vi "MEASure_FETCh_READ.vi"(4 "Timeout (ms)":u32=1000, 5 "Sleep":bool, 6 "Digits":u8=5 min=1 max=5 step=1, 7 "Function":enum16{"MEASure", "READ", "FETCh"}(ring), 8 "Error in (no error)":errorcluster, 9 "Size":u16=1 min=1 max=4096 step=1, 10 "Select":T1={"X"=FALSE, "Y"=TRUE, "Z"=FALSE, "Temp"=FALSE, "Timstamp"=FALSE}, 11 "VISA resource":refnum<visa-resource-name>) -> (0 "Error out":errorcluster, 2 "Output":T2 {"Z" format="%.5f"; "Y" format="%.5f"; "X" format="%.5f"}, 3 "Dup VISA resource":refnum<visa-resource-name>)   [LabVIEW 2010]
doc: "Copyright (c) 2012 Metrolab Technology SA, Plan-les-Ouates, Geneva, Switzerland\nPerforms a measurement and parses the result."
panel:
  # "MEASure_FETCh_READ"
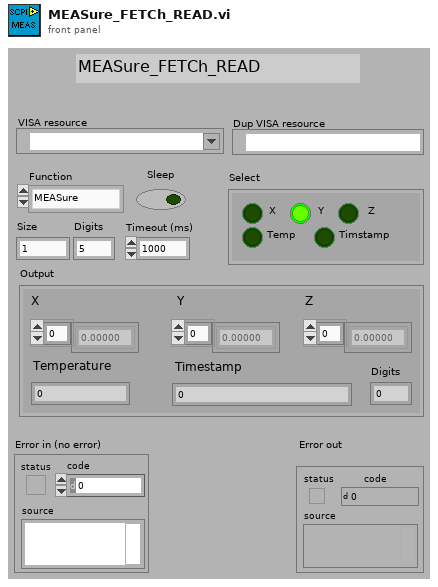
[diagram p1: front panel]
types:
  T1 = cluster{"X":bool, "Y":bool, "Z":bool, "Temp":bool, "Timstamp":bool}
  T2 = cluster{"X":dbl[], "Y":dbl[], "Z":dbl[], "Temperature":u16, "Timestamp":ext, "Digits":u8}
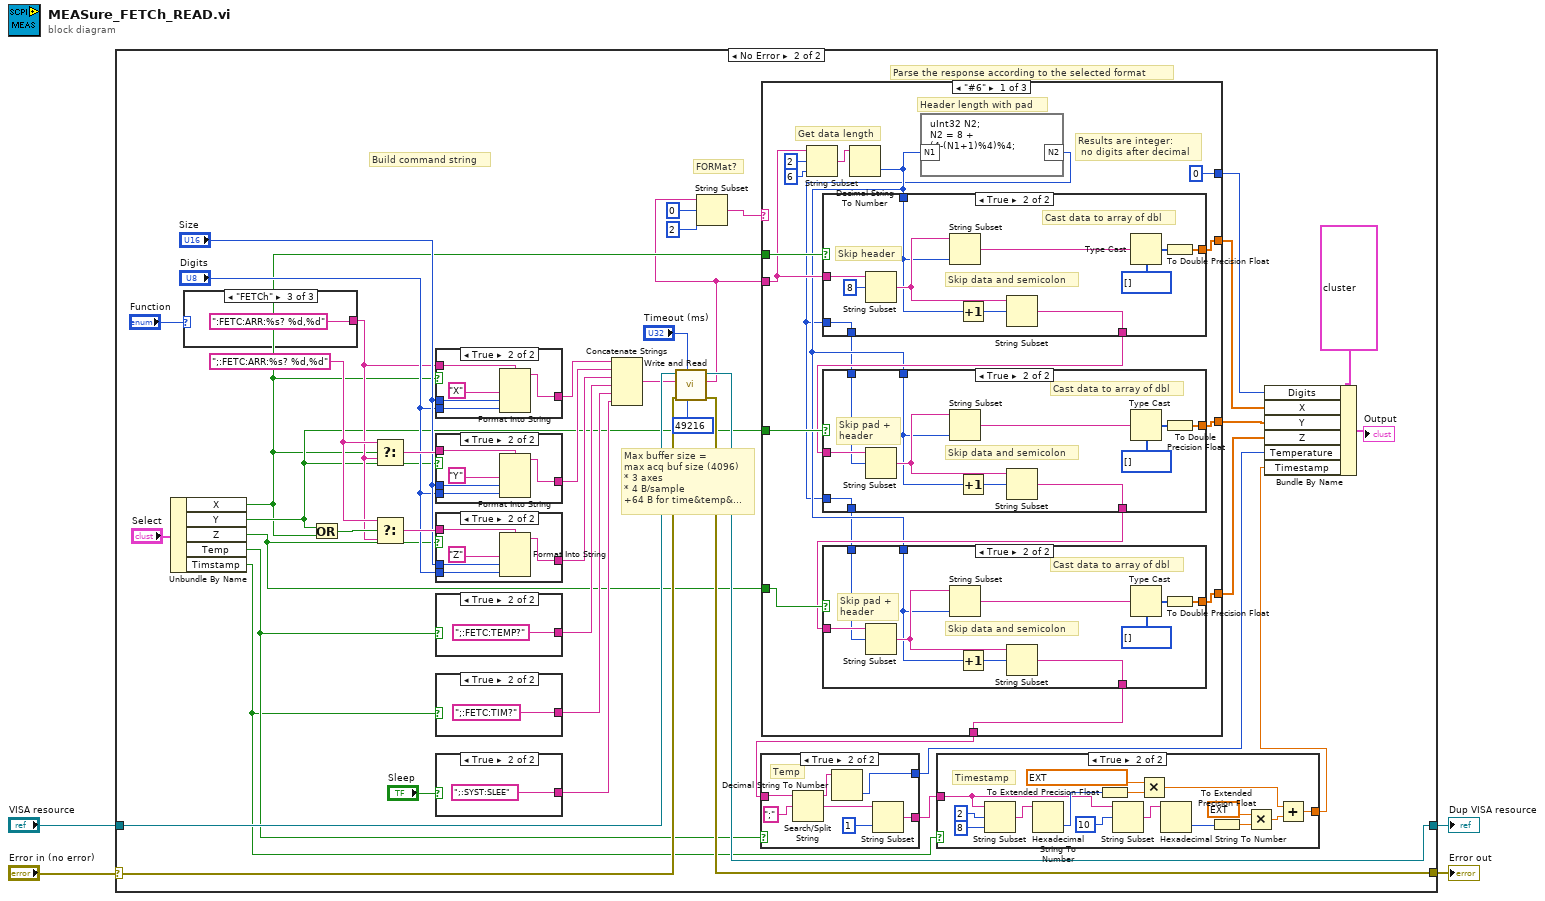
[diagram p0: block diagram]
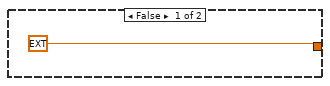
[diagram p3: hidden frame]
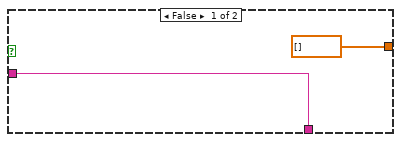
[diagram p4: hidden frame]
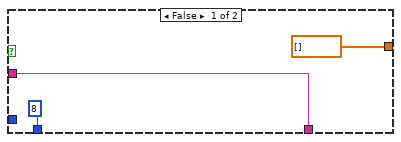
[diagram p5: hidden frame]
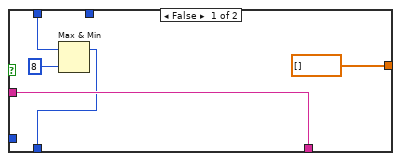
[diagram p6: hidden frame]
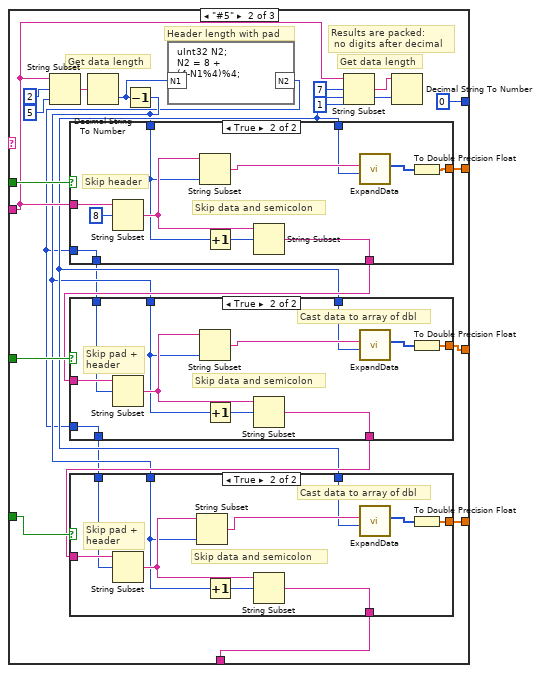
[diagram p7: hidden frame]
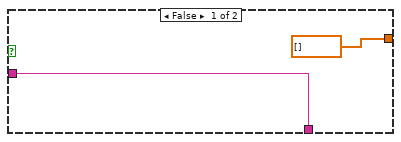
[diagram p8: hidden frame]
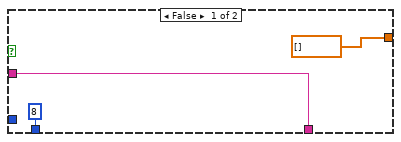
[diagram p9: hidden frame]
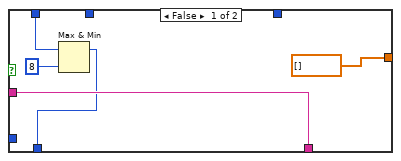
[diagram p10: hidden frame]
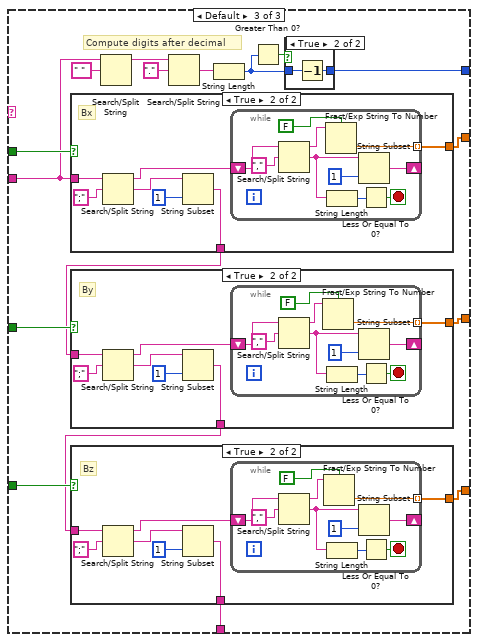
[diagram p11: hidden frame]
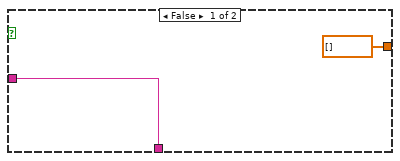
[diagram p13: hidden frame]
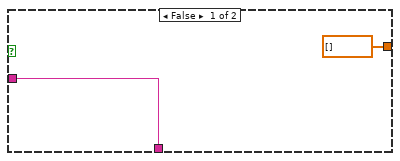
[diagram p14: hidden frame]
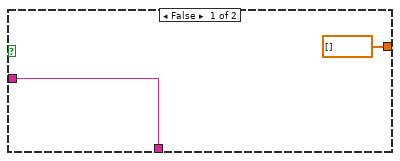
[diagram p15: hidden frame]
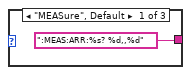
[diagram p16: hidden frame]
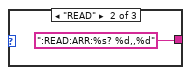
[diagram p17: hidden frame]
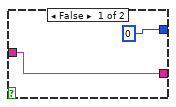
[diagram p18: hidden frame]
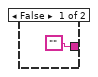
[diagram p19: hidden frame]
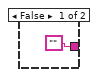
[diagram p20: hidden frame]
diagram:
  n1 = case shown="No Error" "Error in (no error)" {
    selector: "Error in (no error)" -> [w5 w46]
    tunnel: "VISA resource" -> [w6 w47]
    tunnel: [w6 w44] -> w2
    tunnel: [w5 w45] -> w4
    frame Error {
    }
    frame No Error {
      w43 = ";:FETC:ARR:%s? %d,%d"
      # "Max buffer size =\nmax acq buf size (4096)\n* 3 axes\n* 4 B/sample\n+64 B for time&temp&..."
      # "FORMat?"
      # "Parse the response according to the selected format"
      # "Build command string"
      n2 = Unbundle By Name("Select") -> ("X"=w13:bool, "Y"=w15:bool, "Z"=w14:bool, "Temp"=w24:bool, "Timstamp"=w11:bool)
      n3 = case shown="\"FETCh\"" "Function" {
        tunnel: [":MEAS:ARR:%s? %d,,%d" ":READ:ARR:%s? %d,,%d" ":FETC:ARR:%s? %d,%d"] -> w22
        frame "MEASure", Default {
        }
        frame "READ" {
        }
        frame "FETCh" {
        }
      }
      n4 = Or(x=w15, y=w13) -> (x .or. y?=w42:bool)
      n5 = Select(t=w43, s=w13, f=w22) -> (s? t:f=w33:string)
      n6 = Select(t=w43, s=w42, f=w22) -> (s? t:f=w32:string)
      n7 = case shown="True" w13 {
        tunnel: w22 -> [_ w302]
        tunnel: ["" w298] -> w41
        tunnel: "Size" -> [_ w301]
        tunnel: "Digits" -> [_ w299]
        frame False {
        }
        frame True {
          n8 = Format Into String(format string=w302, "X", w301, w299) -> (resulting string=w298:string)  [unwired: 2 in, 1 out]
        }
      }
      n9 = case shown="True" w15 {
        tunnel: w33 -> [_ w290]
        tunnel: ["" w286] -> w29
        tunnel: "Size" -> [_ w289]
        tunnel: "Digits" -> [_ w287]
        frame False {
        }
        frame True {
          n10 = Format Into String(format string=w290, "Y", w289, w287) -> (resulting string=w286:string)  [unwired: 2 in, 1 out]
        }
      }
      n11 = case shown="True" w14 {
        tunnel: w32 -> [_ w284]
        tunnel: ["" w280] -> w30
        tunnel: "Size" -> [_ w283]
        tunnel: "Digits" -> [_ w281]
        frame False {
        }
        frame True {
          n12 = Format Into String(format string=w284, "Z", w283, w281) -> (resulting string=w280:string)  [unwired: 2 in, 1 out]
        }
      }
      n13 = case shown="True" w24 {
        tunnel: ["" ";:FETC:TEMP?"] -> w40
        frame False {
        }
        frame True {
        }
      }
      n14 = case shown="True" w11 {
        tunnel: ["" ";:FETC:TIM?"] -> w39
        frame False {
        }
        frame True {
        }
      }
      n15 = case shown="True" "Sleep" {
        tunnel: ["" ";:SYST:SLEE"] -> w38
        frame False {
        }
        frame True {
        }
      }
      n16 = Concatenate Strings(w41, w29, w30, w40, w39, w38) -> (w37:string)
      n17 = call "Write and Read.vi"("Num bytes"=u32 49216, "Timeout (ms)"="Timeout (ms)", "Error in (no error)"=w46, "Command"=w37, "VISA resource"=w47) -> ("Error out"=w45:errorcluster, "Response"=w12:string, "Dup VISA resource"=w44:refnum<visa-resource-name>)  [unwired: 2 in, 2 out]
      n18 = String Subset(string=w12, offset (0)=0, length (rest)=2 ("length (rest)")) -> (substring=w7:string)
      n19 = case shown="\"#6\"" w7 {
        tunnel: w13 -> [w79 w144 w206]
        tunnel: [w73 w138 w205] -> w19
        tunnel: w15 -> [w80 w145 w204]
        tunnel: w14 -> [w78 w143 w203]
        tunnel: [w74 w139 w201] -> w17
        tunnel: w12 -> [w69 w132 w197]
        tunnel: [0 0 w191] -> w20
        tunnel: [w77 w142 w190] -> w16
        tunnel: [w81 w146 w202] -> w18
        frame "#6" {
          # "Header length with pad"
          # "Get data length"
          # "Results are integer:\n no digits after decimal"
          n20 = String Subset(string=w69, offset (0)=2, length (rest)=6 ("length (rest)")) -> (substring=w72:string)
          n21 = Decimal String To Number(string=w72) -> (number=w68:i32)  [unwired: 2 in, 1 out]
          n22 = formula code="uInt32 N2;\nN2 = 8 +\n(4-(N1+1)%4)%4;"("N1"=w68) -> ("N2"=w65:u32)
          n23 = case shown="True" w79 {
            tunnel: [dbl[] [] w104] -> w73
            tunnel: w69 -> [w97 w103]
            tunnel: [w97 w107] -> w75
            tunnel: w68 -> [_ w100]
            tunnel: [u32 8 ("offset (0)") w98] -> w67
            tunnel: w65 -> [_ w98]
            frame False {
            }
            frame True {
              # "Skip data and semicolon"
              # "Cast data to array of dbl"
              # "Skip header"
              n24 = String Subset(string=w103, offset (0)=8) -> (substring=w101:string)  [unwired: 1 in]
              n25 = String Subset(string=w101, length (rest)=w100) -> (substring=w102:string)  [unwired: 1 in]
              n26 = Increment(x=w100) -> (x+1=w99:i32)
              n27 = String Subset(string=w101, offset (0)=w99) -> (substring=w107:string)  [unwired: 1 in]
              n28 = Type Cast(type=i32[] [], x=w102) -> (*(type *) &x=w105:i32[])
              n29 = To Double Precision Float(number=w105) -> (double precision float=w104:dbl[])
            }
          }
          n30 = case shown="True" w80 {
            tunnel: [dbl[] [] w122] -> w81
            tunnel: w75 -> [w112 w120]
            tunnel: [w112 w121] -> w76
            tunnel: w68 -> [_ w118]
            tunnel: w67 -> [w110 w115]
            tunnel: [w109 w114] -> w66
            tunnel: w65 -> [_ w114]
            frame False {
              n31 = Max & Min(x=w110, y=u32 8 ("offset (0)")) -> (max(x,y)=w109:u32)  [unwired: 1 out]
            }
            frame True {
              # "Skip data and semicolon"
              # "Cast data to array of dbl"
              # "Skip pad + \nheader"
              n32 = String Subset(string=w120, offset (0)=w115) -> (substring=w119:string)  [unwired: 1 in]
              n33 = String Subset(string=w119, length (rest)=w118) -> (substring=w116:string)  [unwired: 1 in]
              n34 = Increment(x=w118) -> (x+1=w117:i32)
              n35 = String Subset(string=w119, offset (0)=w117) -> (substring=w121:string)  [unwired: 1 in]
              n36 = Type Cast(type=i32[] [], x=w116) -> (*(type *) &x=w123:i32[])
              n37 = To Double Precision Float(number=w123) -> (double precision float=w122:dbl[])
            }
          }
          n38 = case shown="True" w78 {
            tunnel: [dbl[] [] w93] -> w74
            tunnel: w76 -> [w83 w91]
            tunnel: [w83 w90] -> w77
            tunnel: w68 -> [_ w87]
            tunnel: w66 -> [_ w85]
            frame False {
            }
            frame True {
              # "Skip data and semicolon"
              # "Cast data to array of dbl"
              # "Skip pad +\nheader"
              n39 = String Subset(string=w91, offset (0)=w85) -> (substring=w89:string)  [unwired: 1 in]
              n40 = String Subset(string=w89, length (rest)=w87) -> (substring=w88:string)  [unwired: 1 in]
              n41 = Increment(x=w87) -> (x+1=w86:i32)
              n42 = String Subset(string=w89, offset (0)=w86) -> (substring=w90:string)  [unwired: 1 in]
              n43 = Type Cast(type=i32[] [], x=w88) -> (*(type *) &x=w92:i32[])
              n44 = To Double Precision Float(number=w92) -> (double precision float=w93:dbl[])
            }
          }
        }
        frame "#5" {
          # "Header length with pad"
          # "Get data length"
          # "Get data length"
          # "Results are packed:\n no digits after decimal"
          n45 = String Subset(string=w132, offset (0)=2, length (rest)=5 ("length (rest)")) -> (substring=w137:string)
          n46 = Decimal String To Number(string=w137) -> (number=w128:i32)  [unwired: 2 in, 1 out]
          n47 = Decrement(x=w128) -> (x-1=w129:i32)
          n48 = formula code="uInt32 N2;\nN2 = 8 +\n(4-N1%4)%4;"("N1"=w128) -> ("N2"=w125:u32)
          n49 = String Subset(string=w132, offset (0)=7, length (rest)=1 ("length (rest)")) -> (substring=w133:string)
          n50 = Decimal String To Number(string=w133) -> (number=w130:i32)  [unwired: 2 in, 1 out]
          n51 = case shown="True" w144 {
            tunnel: [dbl[] [] w172] -> w138
            tunnel: w132 -> [w162 w171]
            tunnel: [w162 w173] -> w140
            tunnel: w129 -> [_ w165]
            tunnel: w130 -> [_ w168]
            tunnel: [u32 8 ("offset (0)") w163] -> w127
            tunnel: w125 -> [_ w163]
            frame False {
            }
            frame True {
              # "Skip data and semicolon"
              # "Skip header"
              n52 = String Subset(string=w171, offset (0)=8) -> (substring=w170:string)  [unwired: 1 in]
              n53 = String Subset(string=w170, length (rest)=w165) -> (substring=w169:string)  [unwired: 1 in]
              n54 = Increment(x=w165) -> (x+1=w164:i32)
              n55 = String Subset(string=w170, offset (0)=w164) -> (substring=w173:string)  [unwired: 1 in]
              n56 = call "ExpandData.vi"("Data length"=w168, "Input"=w169) -> ("Output"=w167:i32[])  [unwired: 8 in]
              n57 = To Double Precision Float(number=w167) -> (double precision float=w172:dbl[])
            }
          }
          n58 = case shown="True" w145 {
            tunnel: [dbl[] [] w189] -> w146
            tunnel: w140 -> [w177 w187]
            tunnel: [w177 w188] -> w141
            tunnel: w129 -> [_ w182]
            tunnel: w130 -> [_ w184]
            tunnel: w127 -> [w175 w180]
            tunnel: [w174 w179] -> w126
            tunnel: w125 -> [_ w179]
            frame False {
              n59 = Max & Min(x=w175, y=u32 8 ("offset (0)")) -> (max(x,y)=w174:u32)  [unwired: 1 out]
            }
            frame True {
              # "Skip data and semicolon"
              # "Cast data to array of dbl"
              # "Skip pad +\nheader"
              n60 = String Subset(string=w187, offset (0)=w180) -> (substring=w186:string)  [unwired: 1 in]
              n61 = String Subset(string=w186, length (rest)=w182) -> (substring=w185:string)  [unwired: 1 in]
              n62 = Increment(x=w182) -> (x+1=w181:i32)
              n63 = String Subset(string=w186, offset (0)=w181) -> (substring=w188:string)  [unwired: 1 in]
              n64 = call "ExpandData.vi"("Data length"=w184, "Input"=w185) -> ("Output"=w183:i32[])  [unwired: 8 in]
              n65 = To Double Precision Float(number=w183) -> (double precision float=w189:dbl[])
            }
          }
          n66 = case shown="True" w143 {
            tunnel: [dbl[] [] w159] -> w139
            tunnel: w141 -> [w148 w158]
            tunnel: [w148 w157] -> w142
            tunnel: w129 -> [_ w155]
            tunnel: w130 -> [_ w151]
            tunnel: w126 -> [_ w150]
            frame False {
            }
            frame True {
              # "Skip pad +\nheader"
              # "Skip data and semicolon"
              # "Cast data to array of dbl"
              n67 = String Subset(string=w158, offset (0)=w150) -> (substring=w156:string)  [unwired: 1 in]
              n68 = String Subset(string=w156, length (rest)=w155) -> (substring=w152:string)  [unwired: 1 in]
              n69 = Increment(x=w155) -> (x+1=w154:i32)
              n70 = String Subset(string=w156, offset (0)=w154) -> (substring=w157:string)  [unwired: 1 in]
              n71 = call "ExpandData.vi"("Data length"=w151, "Input"=w152) -> ("Output"=w153:i32[])  [unwired: 8 in]
              n72 = To Double Precision Float(number=w153) -> (double precision float=w159:dbl[])
            }
          }
        }
        frame Default {
          # "Compute digits after decimal"
          n73 = case shown="True" w206 {
            tunnel: w197 -> [w249 w252]
            tunnel: [w249 w251] -> w200
            tunnel: [dbl[] [] w250] -> w205
            frame False {
            }
            frame True {
              # "Bx"
              n74 = Search/Split String(string=w252, search string/char (-)=";") -> (substring before match=w253:string, match + rest of string=w254:string)  [unwired: 1 in, 1 out]
              n75 = String Subset(string=w254, offset (0)=1) -> (substring=w251:string)  [unwired: 1 in]
              n76 = while {
                shift-right: [w263] -> _
                shift-left: w253 -> [w265]
                tunnel: [w258] -> w250 mode=indexing
                stop <- w260 stop-if-true
                n77 = Search/Split String(string=w265, search string/char (-)=",") -> (substring before match=w259:string, match + rest of string=w262:string)  [unwired: 1 in, 1 out]
                n78 = Fract/Exp String To Number(use system decimal point (T)=FALSE, string=w259) -> (number=w258:dbl)  [unwired: 2 in, 1 out]
                n79 = String Length(string=w262) -> (length=w261:i32)
                n80 = String Subset(string=w262, offset (0)=1) -> (substring=w263:string)  [unwired: 1 in]
                n81 = Less Or Equal To 0?(x=w261) -> (x <= 0?=w260:bool)
              }
            }
          }
          n82 = case shown="True" w204 {
            tunnel: w200 -> [w230 w233]
            tunnel: [w230 w232] -> w199
            tunnel: [dbl[] [] w231] -> w202
            frame False {
            }
            frame True {
              # "By"
              n83 = Search/Split String(string=w233, search string/char (-)=";") -> (substring before match=w234:string, match + rest of string=w235:string)  [unwired: 1 in, 1 out]
              n84 = String Subset(string=w235, offset (0)=1) -> (substring=w232:string)  [unwired: 1 in]
              n85 = while {
                shift-right: [w244] -> _
                shift-left: w234 -> [w246]
                tunnel: [w239] -> w231 mode=indexing
                stop <- w241 stop-if-true
                n86 = Search/Split String(string=w246, search string/char (-)=",") -> (substring before match=w240:string, match + rest of string=w243:string)  [unwired: 1 in, 1 out]
                n87 = Fract/Exp String To Number(use system decimal point (T)=FALSE, string=w240) -> (number=w239:dbl)  [unwired: 2 in, 1 out]
                n88 = String Length(string=w243) -> (length=w242:i32)
                n89 = String Subset(string=w243, offset (0)=1) -> (substring=w244:string)  [unwired: 1 in]
                n90 = Less Or Equal To 0?(x=w242) -> (x <= 0?=w241:bool)
              }
            }
          }
          n91 = case shown="True" w203 {
            tunnel: w199 -> [w211 w214]
            tunnel: [w211 w213] -> w190
            tunnel: [dbl[] [] w212] -> w201
            frame False {
            }
            frame True {
              # "Bz"
              n92 = Search/Split String(string=w214, search string/char (-)=";") -> (substring before match=w215:string, match + rest of string=w216:string)  [unwired: 1 in, 1 out]
              n93 = String Subset(string=w216, offset (0)=1) -> (substring=w213:string)  [unwired: 1 in]
              n94 = while {
                shift-right: [w225] -> _
                shift-left: w215 -> [w227]
                tunnel: [w220] -> w212 mode=indexing
                stop <- w222 stop-if-true
                n95 = Search/Split String(string=w227, search string/char (-)=",") -> (substring before match=w221:string, match + rest of string=w224:string)  [unwired: 1 in, 1 out]
                n96 = Fract/Exp String To Number(use system decimal point (T)=FALSE, string=w221) -> (number=w220:dbl)  [unwired: 2 in, 1 out]
                n97 = String Length(string=w224) -> (length=w223:i32)
                n98 = String Subset(string=w224, offset (0)=1) -> (substring=w225:string)  [unwired: 1 in]
                n99 = Less Or Equal To 0?(x=w223) -> (x <= 0?=w222:bool)
              }
            }
          }
          n100 = Search/Split String(string=w197, search string/char (-)=" ") -> (substring before match=w196:string)  [unwired: 1 in, 2 out]
          n101 = Search/Split String(string=w196, search string/char (-)=".") -> (match + rest of string=w194:string)  [unwired: 1 in, 2 out]
          n102 = String Length(string=w194) -> (length=w193:i32)
          n103 = Greater Than 0?(x=w193) -> (x > 0?=w192:bool)
          n104 = case shown="True" w192 {
            tunnel: w193 -> [w207 w209]
            tunnel: [w207 w208] -> w191
            frame False {
            }
            frame True {
              n105 = Decrement(x=w209) -> (x-1=w208:i32)
            }
          }
        }
      }
      n106 = case shown="True" w24 {
        tunnel: [w270 w275] -> w10
        tunnel: [0 w273] -> w25
        tunnel: w16 -> [w270 w272]
        frame False {
        }
        frame True {
          # "Temp"
          n107 = Search/Split String(string=w272, search string/char (-)=";") -> (substring before match=w274:string, match + rest of string=w276:string)  [unwired: 1 in, 1 out]
          n108 = Decimal String To Number(string=w274) -> (number=w273:i32)  [unwired: 2 in, 1 out]
          n109 = String Subset(string=w276, offset (0)=1) -> (substring=w275:string)  [unwired: 1 in]
        }
      }
      n110 = case shown="True" w11 {
        tunnel: w10 -> [_ w56]
        tunnel: [ext 0.0 w51] -> w8
        frame False {
        }
        frame True {
          # "Timestamp"
          n111 = String Subset(string=w56, offset (0)=2 ("offset"), length (rest)=8 ("length (rest)")) -> (substring=w59:string)
          n112 = Hexadecimal String To Number(string=w59) -> (number=w64:u32)  [unwired: 2 in, 1 out]
          n113 = To Extended Precision Float(1:w64) -> (0:w63:ext)
          n114 = String Subset(string=w56, offset (0)=10 ("offset")) -> (substring=w58:string)  [unwired: 1 in]
          n115 = Multiply(x=ext 4.294967296 ("y"), y=w63) -> (x*y=w50:ext)
          n116 = Hexadecimal String To Number(string=w58) -> (number=w54:u32)  [unwired: 2 in, 1 out]
          n117 = To Extended Precision Float(1:w54) -> (0:w55:ext)
          n118 = Multiply(x=ext 1e-9 ("y"), y=w55) -> (x*y=w52:ext)
          n119 = Add(x=w50, y=w52) -> (x+y=w51:ext)
        }
      }
      n120 = Bundle By Name(cluster=T2 {"X"=[], "Y"=[0.0106], "Z"=[], "Temperature"=0, "Timestamp"=0.0, "Digits"=5} ("Output"), "Digits"=w20, "X"=w19, "Y"=w18, "Z"=w17, "Temperature"=w25, "Timestamp"=w8) -> (→"Output":T2)
    }
  }
  "Error out" <- w4
  "Dup VISA resource" <- w2
